vi "update dbc.vi"(8 "error in (no error)":errorcluster, 11 "Boolean":bool=TRUE) -> (0 "error out":errorcluster)   [LabVIEW 2018]
uses:
  <vilib>/xnet/xnet.llb/XNET Frame CAN.ctl
  <vilib>/xnet/xnet.llb/XNET Frame Type CAN.ctl
  <vilib>/xnet/xnet.llb/XNET Create Session (Frame Output Single-point).vi
  <vilib>/xnet/xnet.llb/XNET Write (Frame CAN).vi
  <resource>/objmgr/xnet.rc
panel:
  out "Frames":refnum<k21>[](array[refnum])
  out "array of alias":string[](array[string])
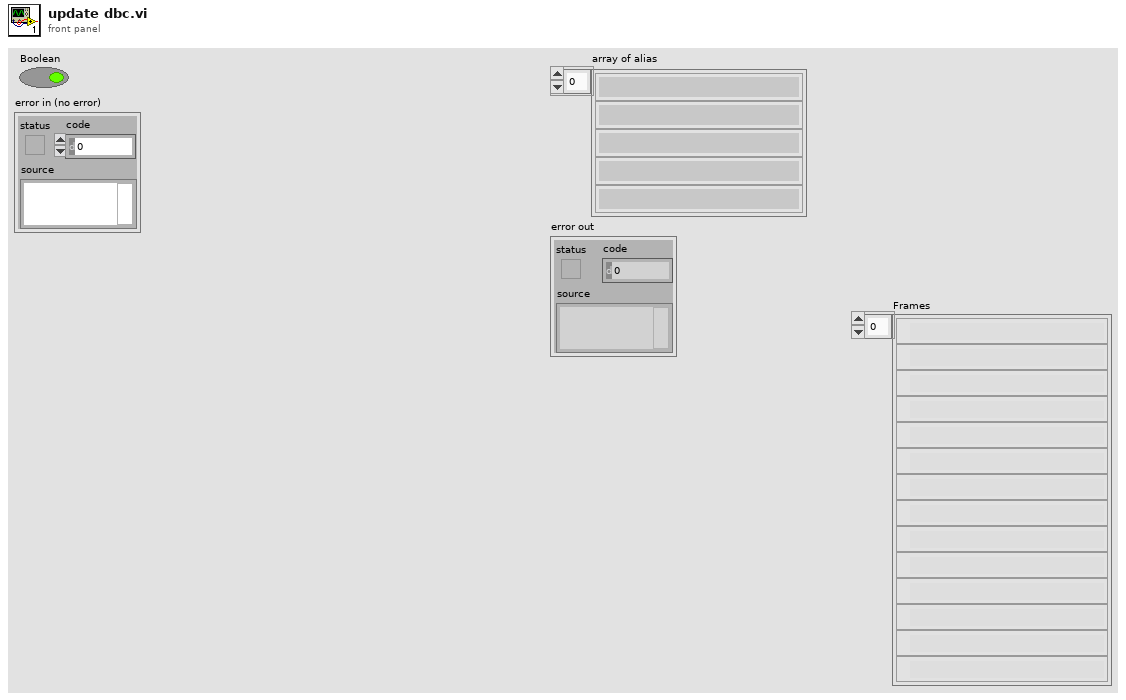
[diagram p1: front panel]
types:
  T1 = typedef "XNET Frame CAN.ctl" = cluster{"timestamp":timestamp, "payload":u8[], "identifier":u32, "type":T2, "extended?":bool, "echo?":bool}
  T2 = typedef "XNET Frame Type CAN.ctl" = u8
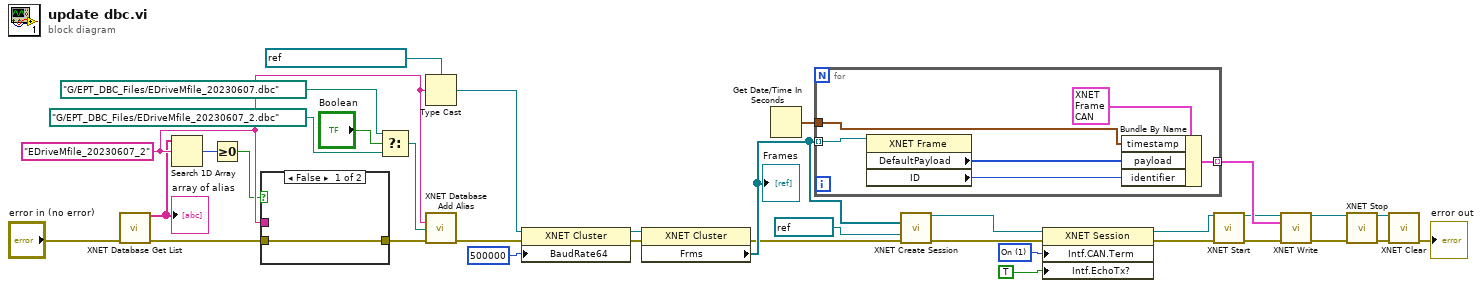
[diagram p0: block diagram]
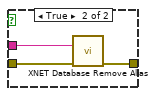
[diagram p2: hidden frame]
diagram:
  w16 = u32 1 items=["Off", "On"] ("Interface:CAN:Termination")
  w35 = "EDriveMfile_20230607_2" ("element")
  n1 = call <vilib>:"XNET Database Get List.vi"("error in (no error)"="error in (no error)") -> ("array of alias"=w31:string[], "error out"=w29:errorcluster)  [unwired: 12 in, 1 out]
  "array of alias" <- w31
  n2 = Search 1D Array(1D array=w31, element=w35) -> (index of element=w30:i32)  [unwired: 1 in]
  n3 = Greater Or Equal To 0?(x=w30) -> (x >= 0?=w28:bool)
  n4 = case shown="False" w28 {
    tunnel: w29 -> [w36 w39]
    tunnel: w35 -> [_ w38]
    tunnel: [w36 w37] -> w23
    frame False {
    }
    frame True {
      n5 = call <vilib>:"XNET Database Remove Alias.vi"("alias"=w38, "error in (no error)"=w39) -> ("error out"=w37:errorcluster)  [unwired: 13 in]
    }
  }
  n6 = Select(t=path "G:/EPT_DBC_Files/EDriveMfile_20230607.dbc" ("filepath"), s="Boolean", f=path "G:/EPT_DBC_Files/EDriveMfile_20230607_2.dbc") -> (s? t:f=w26:path)
  n7 = Type Cast(type=refnum<k21> "EDriveMfile_20230607" ("XNET Cluster"), x=w35) -> (*(type *) &x=w33:refnum<k21>)
  n8 = call <vilib>:"XNET Database Add Alias.vi"("alias"=w35, "filepath"=w26, "error in (no error)"=w23) -> ("error out"=w21:errorcluster)  [unwired: 12 in]
  n9 = property class="XNET Cluster"(reference=w33, error in=w21, "BaudRate64"=u64 500000 ("64bit Baud Rate")) -> (reference out=w12:refnum<k21>, error out=w11:errorcluster)
  n10 = property class="XNET Cluster"(reference=w12, error in=w11) -> (error out=w10:errorcluster, "Frms"=w19:refnum<k21>[])  [unwired: 1 out]
  "Frames" <- w19
  n11 = Get Date/Time In Seconds() -> (seconds since 1Jan1904=w13:timestamp)
  n12 = for {
    tunnel: w19 -> [w45] mode=indexing
    tunnel: [w41] -> w18 mode=indexing
    tunnel: w13 -> [w40]
    n13 = property class="XNET Frame"(reference=w45) -> ("DefaultPayload"=w42:u8[], "ID"=w43:u32)  [unwired: 1 in, 2 out]
    n14 = Bundle By Name(cluster=T1 {"timestamp"=timestamp(0 s since 1904-01-01), "payload"=[], "identifier"=0, "type"=0, "extended?"=FALSE, "echo?"=FALSE} ("CAN frame"), "timestamp"=w40, "payload"=w42, "identifier"=w43) -> (w41:T1)
  }
  n15 = call-poly <vilib>:"XNET Create Session.vi"("frame list"=w19, "interface"=refnum<k21> "CAN1", "error in (no error)"=w10) -> ("session out"=w17:refnum<k21>, "error out"=w14:errorcluster)  [unwired: 11 in]
  n16 = property class="XNET Session"(reference=w17, error in=w14, "Intf.CAN.Term"=w16, "Intf.EchoTx?"=TRUE ("Interface:Echo Transmit?")) -> (reference out=w7:refnum<k21>, error out=w6:errorcluster)
  n17 = call <vilib>:"XNET Start.vi"("session in"=w7, "error in (no error)"=w6) -> ("session out"=w2:refnum<k21>, "error out"=w5:errorcluster)  [unwired: 12 in]
  n18 = call-poly <vilib>:"XNET Write.vi"("session in"=w2, "data"=w18, "error in (no error)"=w5) -> ("session out"=w3:refnum<k21>, "error out"=w4:errorcluster)  [unwired: 11 in]
  n19 = call <vilib>:"XNET Stop.vi"("session in"=w3, "error in (no error)"=w4) -> ("session out"=w9:refnum<k21>, "error out"=w8:errorcluster)  [unwired: 12 in]
  n20 = call <vilib>:"XNET Clear.vi"("session in"=w9, "error in (no error)"=w8) -> ("error out"=→"error out":errorcluster)  [unwired: 13 in]
